vi "MPS HV PS Manager.vi"(6 "Model (MPS5)":u8(ring)=53 format="%2x" items=["MPS0.6"=49, "MPS1"=50, "MPS2"=51, "MPS3"=52, "MPS5"=53, "MPS10"=54, "MPS15"=55, "MPS20"=56, "MPS30"=57, "MPS2.5"=97], 7 "Command":T1(ring)=enum."Set Output Voltage", 8 "error in":errorcluster, 9 "Address":u8(ring)=49 format="%2x" items=["0 (Broadcast)"=0, "1"=49, "2"=50, "3"=51, "4"=52, "5"=53, "6"=54, "7"=55, "8"=56], 10 "Output Voltage (V)":dbl=500.0 format="%.1f", 11 "VISA Name":refnum<visa-resource-name>) -> (0 "error out":errorcluster, 1 "ID Address":u8(ring) items=["0"=0, "1"=49, "2"=50, "3"=51, "4"=52, "5"=53, "6"=54, "7"=55, "8"=56], 2 "Current Monitor (uA)":dbl, 3 "Voltage Monitor (V)":dbl)   [LabVIEW 2025]
uses:
  <vilib>/Instr/_visa.llb/VISA Configure Serial Port (Instr).vi
panel:
  out "RX String":string
  out "TX String":string
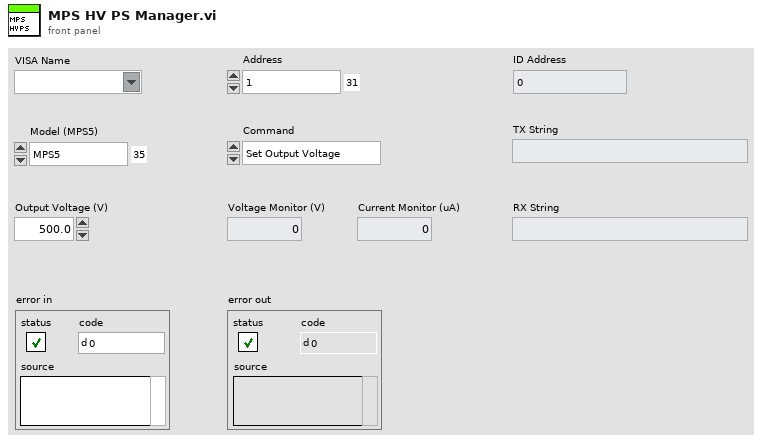
[diagram p1: front panel]
types:
  T1 = enum16{"Init", "Set Output Voltage", "Read Voltage Monitor", "Read Current Monitor", "Disable All", "Enable All", "Read Address", "Set Address", "Close"}
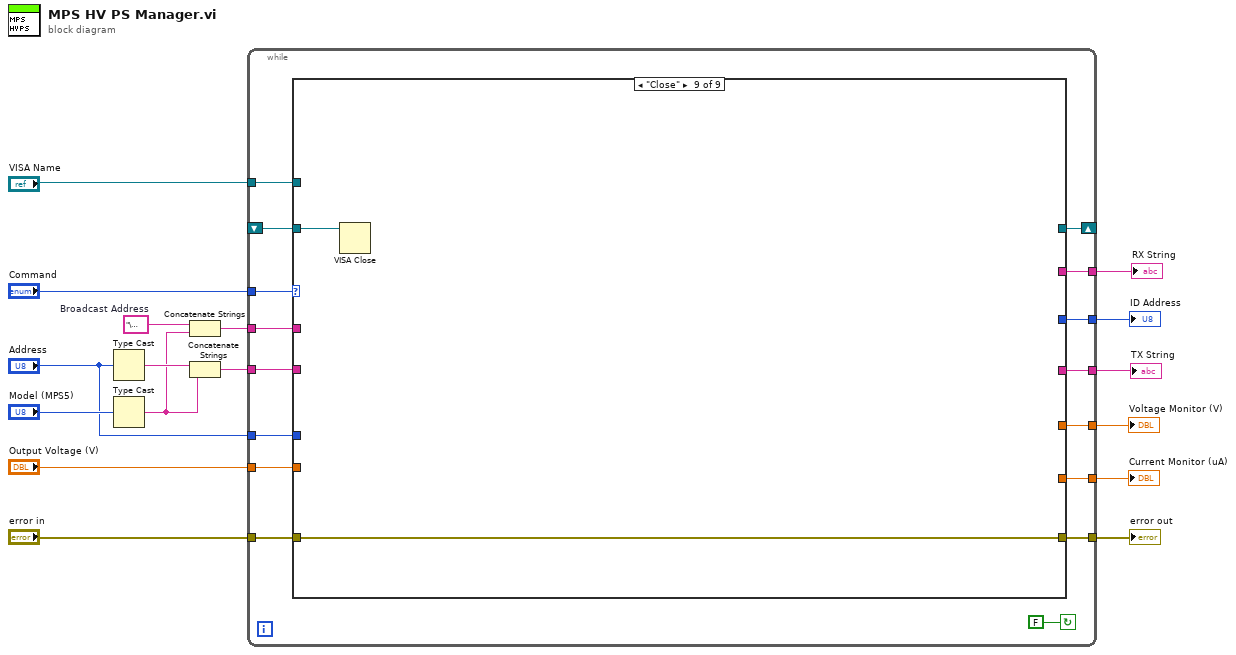
[diagram p0: block diagram]
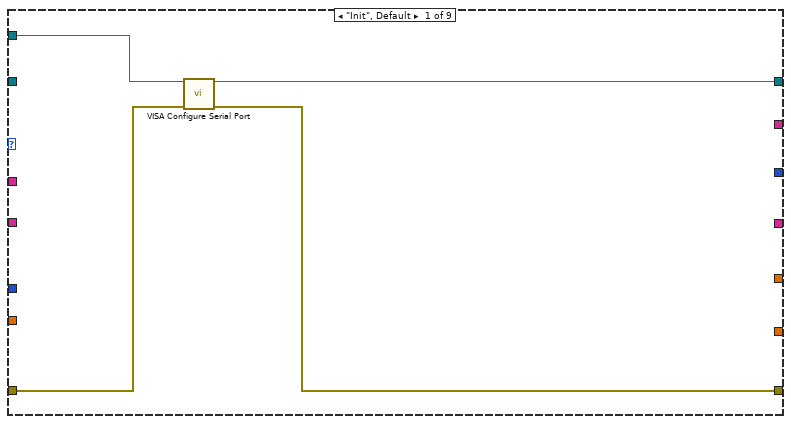
[diagram p2: hidden frame]
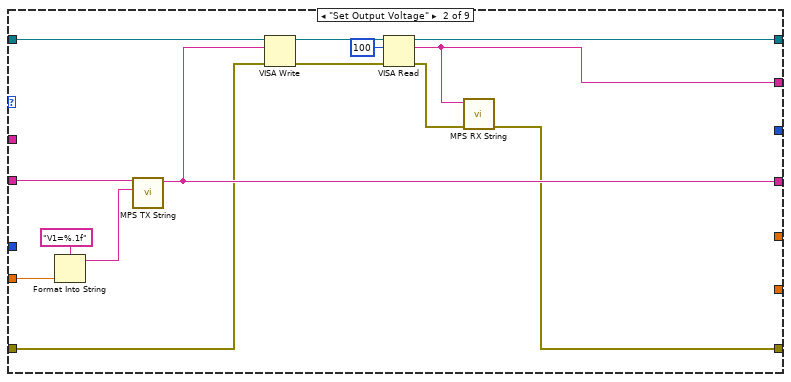
[diagram p3: hidden frame]
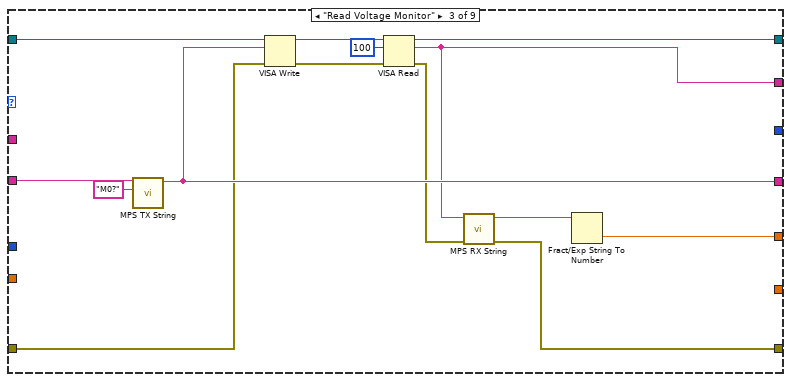
[diagram p4: hidden frame]
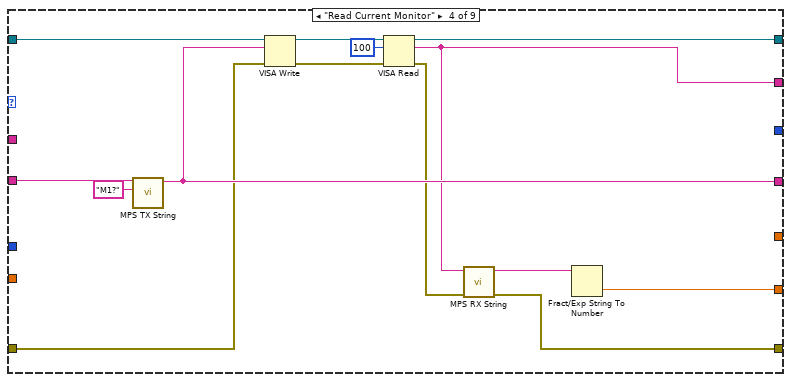
[diagram p5: hidden frame]
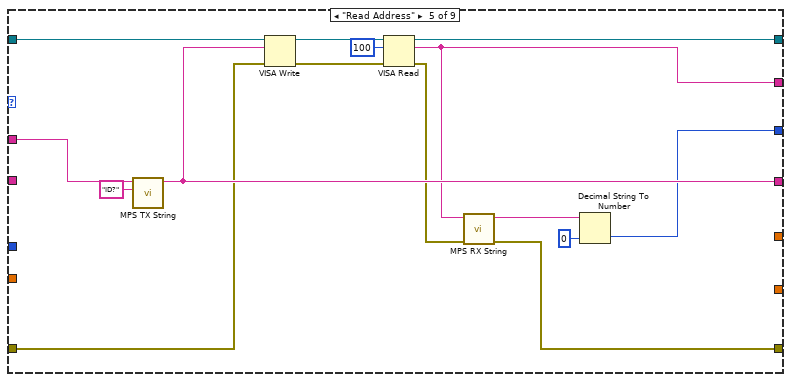
[diagram p6: hidden frame]
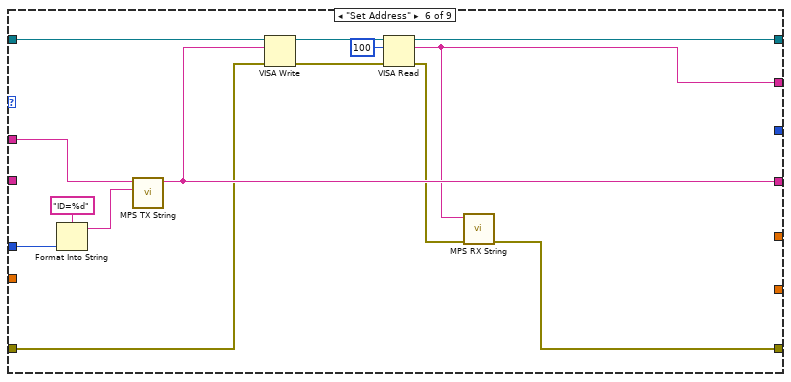
[diagram p7: hidden frame]
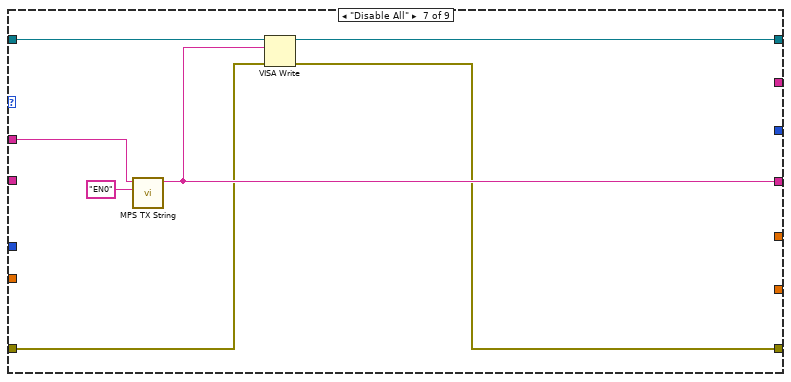
[diagram p8: hidden frame]
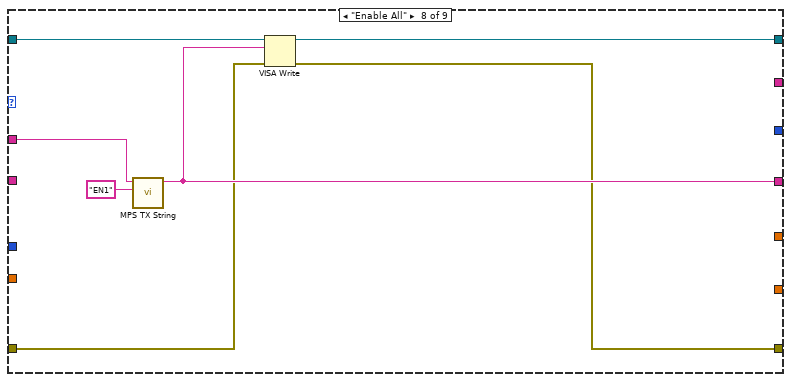
[diagram p9: hidden frame]
diagram:
  w4 = "\u0000"  # Broadcast Address
  n1 = Type Cast(x="Address") -> (*(type *) &x=w12:string)  [unwired: 1 in]
  n2 = Type Cast(x="Model (MPS5)") -> (*(type *) &x=w5:string)  [unwired: 1 in]
  n3 = Concatenate Strings(w4, w5) -> (w3:string)
  n4 = Concatenate Strings(w12, w5) -> (w11:string)
  n5 = while {
    tunnel: "Command" -> [w33]
    tunnel: "VISA Name" -> [w31]
    shift-right: [w30] -> _
    shift-left: _ -> [w29]
    tunnel: "error in" -> [w28]
    tunnel: "Output Voltage (V)" -> [w27]
    tunnel: w11 -> [w26]
    tunnel: [w25] -> w10
    tunnel: [w24] -> w9
    tunnel: [w23] -> w8
    tunnel: [w22] -> w7
    tunnel: [w21] -> w6
    tunnel: w3 -> [w20]
    tunnel: [w19] -> w2
    tunnel: "Address" -> [w18]
    stop <- FALSE continue-if-true
    n6 = case shown="\"Close\"" w33 {
      tunnel: w31 -> [w37 _ _ _ _ _ _ _ _]
      tunnel: [w36 w44 w61 w75 w91 w105 w113 w120 _] -> w30
      tunnel: w29 -> [_ w47 w64 w78 w94 w108 w115 w122 w124]
      tunnel: w28 -> [w35 w41 w58 w72 w88 w102 w112 w119 w123]
      tunnel: w27 -> [_ w50 _ _ _ _ _ _ _]
      tunnel: w26 -> [_ w51 w65 w79 _ _ _ _ _]
      tunnel: [_ w46 w63 w77 w93 w107 w114 w121 _] -> w25
      tunnel: [_ w40 w57 w71 w87 w101 _ _ _] -> w24
      tunnel: [w34 w38 w55 w69 w85 w99 w109 w116 w123] -> w23
      tunnel: [_ _ w52 _ _ _ _ _ _] -> w22
      tunnel: [_ _ _ w66 _ _ _ _ _] -> w21
      tunnel: w20 -> [_ _ _ _ w82 w98 w110 w117 _]
      tunnel: [_ _ _ _ w81 _ _ _ _] -> w19
      tunnel: w18 -> [_ _ _ _ _ w96 _ _ _]
      frame "Init", Default {
        n7 = call-poly "VISA Configure Serial Port"("VISA resource name"=w37, "error in (no error)"=w35) -> ("VISA resource name out"=w36:refnum<visa-resource-name>, "error out"=w34:errorcluster)  [unwired: 12 in]
      }
      frame "Set Output Voltage" {
        n8 = Format Into String(format string="V1=%.1f", w50) -> (resulting string=w48:string)  [unwired: 2 in, 1 out]
        n9 = call "MPS TX String.vi"("Command"=w48, "Header"=w51) -> ("TX Out"=w46:string)  [unwired: 9 in]
        n10 = VISA Write(VISA resource name=w47, write buffer=w46, error in (no error)=w41) -> (VISA resource name out=w45:refnum<visa-resource-name>, error out=w42:errorcluster)  [unwired: 1 out]
        n11 = VISA Read(VISA resource name=w45, byte count=u32 100, error in (no error)=w42) -> (VISA resource name out=w44:refnum<visa-resource-name>, read buffer=w40:string, error out=w39:errorcluster)  [unwired: 1 out]
        n12 = call "MPS RX String.vi"("error in"=w39, "RX In"=w40) -> ("error out"=w38:errorcluster)  [unwired: 7 in, 2 out]
      }
      frame "Read Voltage Monitor" {
        n13 = call "MPS TX String.vi"("Command"="M0?", "Header"=w65) -> ("TX Out"=w63:string)  [unwired: 9 in]
        n14 = VISA Write(VISA resource name=w64, write buffer=w63, error in (no error)=w58) -> (VISA resource name out=w62:refnum<visa-resource-name>, error out=w59:errorcluster)  [unwired: 1 out]
        n15 = VISA Read(VISA resource name=w62, byte count=u32 100, error in (no error)=w59) -> (VISA resource name out=w61:refnum<visa-resource-name>, read buffer=w57:string, error out=w56:errorcluster)  [unwired: 1 out]
        n16 = call "MPS RX String.vi"("error in"=w56, "RX In"=w57) -> ("error out"=w55:errorcluster, "Response"=w53:string)  [unwired: 7 in, 1 out]
        n17 = Fract/Exp String To Number(string=w53) -> (number=w52:dbl)  [unwired: 3 in, 1 out]
      }
      frame "Read Current Monitor" {
        n18 = call "MPS TX String.vi"("Command"="M1?", "Header"=w79) -> ("TX Out"=w77:string)  [unwired: 9 in]
        n19 = VISA Write(VISA resource name=w78, write buffer=w77, error in (no error)=w72) -> (VISA resource name out=w76:refnum<visa-resource-name>, error out=w73:errorcluster)  [unwired: 1 out]
        n20 = VISA Read(VISA resource name=w76, byte count=u32 100, error in (no error)=w73) -> (VISA resource name out=w75:refnum<visa-resource-name>, read buffer=w71:string, error out=w70:errorcluster)  [unwired: 1 out]
        n21 = call "MPS RX String.vi"("error in"=w70, "RX In"=w71) -> ("error out"=w69:errorcluster, "Response"=w67:string)  [unwired: 7 in, 1 out]
        n22 = Fract/Exp String To Number(string=w67) -> (number=w66:dbl)  [unwired: 3 in, 1 out]
      }
      frame "Read Address" {
        n23 = call "MPS TX String.vi"("Command"="ID?", "Header"=w82) -> ("TX Out"=w93:string)  [unwired: 9 in]
        n24 = VISA Write(VISA resource name=w94, write buffer=w93, error in (no error)=w88) -> (VISA resource name out=w92:refnum<visa-resource-name>, error out=w89:errorcluster)  [unwired: 1 out]
        n25 = VISA Read(VISA resource name=w92, byte count=u32 100, error in (no error)=w89) -> (VISA resource name out=w91:refnum<visa-resource-name>, read buffer=w87:string, error out=w86:errorcluster)  [unwired: 1 out]
        n26 = call "MPS RX String.vi"("error in"=w86, "RX In"=w87) -> ("error out"=w85:errorcluster, "Response"=w83:string)  [unwired: 7 in, 1 out]
        n27 = Decimal String To Number(string=w83, default (0L)=u8 0 ("default (0 I32)")) -> (number=w81:u8)  [unwired: 1 in, 1 out]
      }
      frame "Set Address" {
        n28 = Format Into String(format string="ID=%d", w96) -> (resulting string=w95:string)  [unwired: 2 in, 1 out]
        n29 = call "MPS TX String.vi"("Command"=w95, "Header"=w98) -> ("TX Out"=w107:string)  [unwired: 9 in]
        n30 = VISA Write(VISA resource name=w108, write buffer=w107, error in (no error)=w102) -> (VISA resource name out=w106:refnum<visa-resource-name>, error out=w103:errorcluster)  [unwired: 1 out]
        n31 = VISA Read(VISA resource name=w106, byte count=u32 100, error in (no error)=w103) -> (VISA resource name out=w105:refnum<visa-resource-name>, read buffer=w101:string, error out=w100:errorcluster)  [unwired: 1 out]
        n32 = call "MPS RX String.vi"("error in"=w100, "RX In"=w101) -> ("error out"=w99:errorcluster)  [unwired: 7 in, 2 out]
      }
      frame "Disable All" {
        n33 = call "MPS TX String.vi"("Command"="EN0", "Header"=w110) -> ("TX Out"=w114:string)  [unwired: 9 in]
        n34 = VISA Write(VISA resource name=w115, write buffer=w114, error in (no error)=w112) -> (VISA resource name out=w113:refnum<visa-resource-name>, error out=w109:errorcluster)  [unwired: 1 out]
      }
      frame "Enable All" {
        n35 = call "MPS TX String.vi"("Command"="EN1", "Header"=w117) -> ("TX Out"=w121:string)  [unwired: 9 in]
        n36 = VISA Write(VISA resource name=w122, write buffer=w121, error in (no error)=w119) -> (VISA resource name out=w120:refnum<visa-resource-name>, error out=w116:errorcluster)  [unwired: 1 out]
      }
      frame "Close" {
        n37 = VISA Close(VISA resource name=w124) -> ()  [unwired: 1 in, 1 out]
      }
    }
  }
  "error out" <- w8
  "Voltage Monitor (V)" <- w7
  "Current Monitor (uA)" <- w6
  "TX String" <- w10
  "RX String" <- w9
  "ID Address" <- w2
